vi "create channel offsets.vi"(7 "channelControl":T1(array[cluster]), 8 "offsets in":dbl[](array[numeric]), 9 "Offset to value:":dbl, 10 "Channel to match:":u16, 11 "Offset type:":T2(ring)) -> (0 "offsets out":dbl[](array[numeric]), 4 "updatedChannels":T1(array[cluster]))   [LabVIEW 2018]
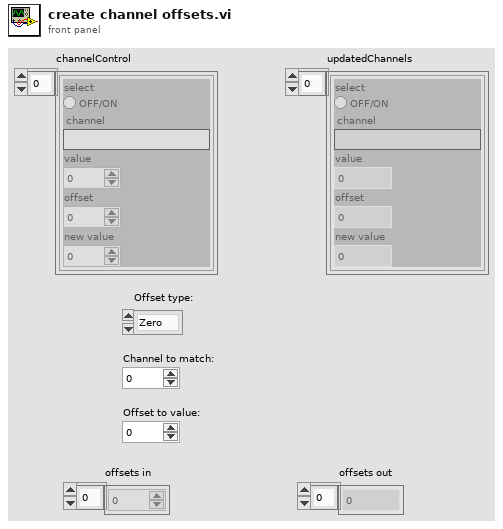
[diagram p1: front panel]
types:
  T1 = cluster{"select":bool, "channel":string, "value":dbl, "offset":dbl, "new value":dbl}[]
  T2 = enum16{"Zero", "Offset to value", "Offset to match channel", "Remove offset"}
  T3 = cluster{"select":bool, "channel":string, "value":dbl, "offset":dbl, "new value":dbl}
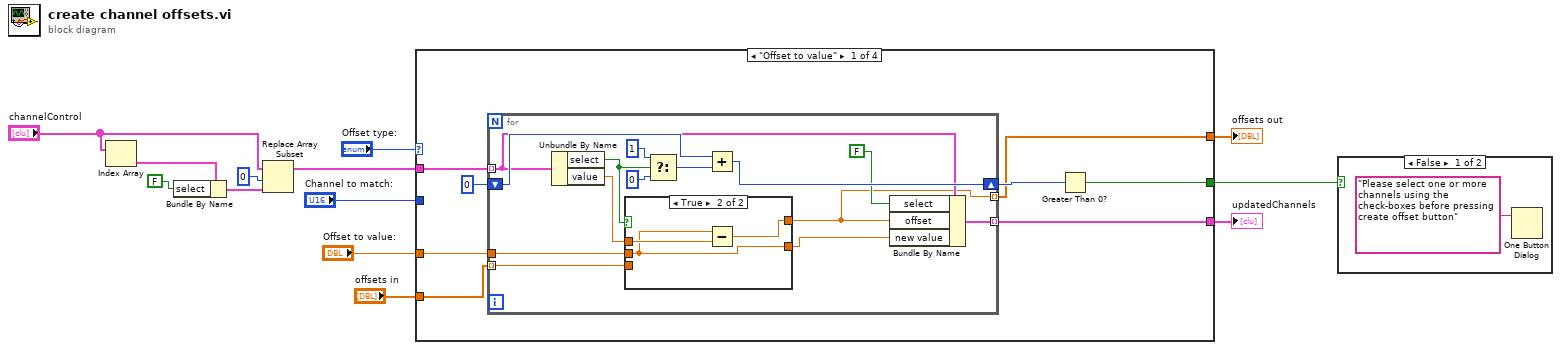
[diagram p0: block diagram]
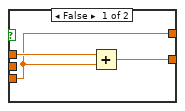
[diagram p3: hidden frame]
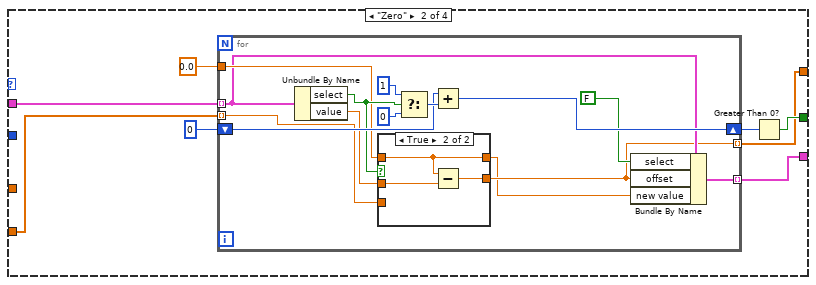
[diagram p4: hidden frame]
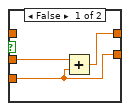
[diagram p5: hidden frame]
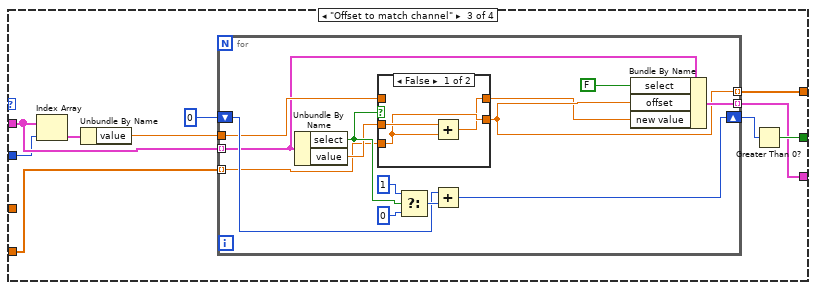
[diagram p6: hidden frame]
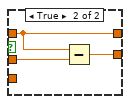
[diagram p7: hidden frame]
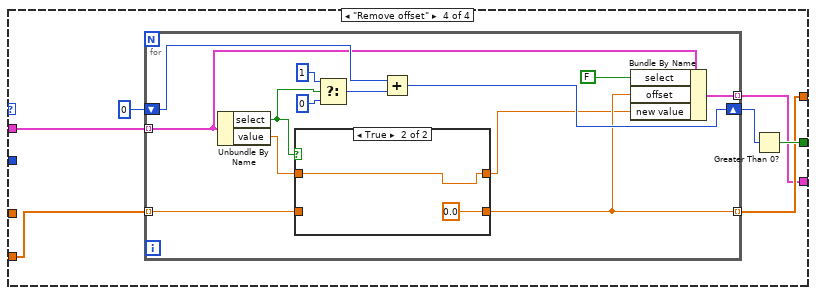
[diagram p8: hidden frame]
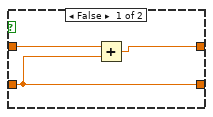
[diagram p9: hidden frame]
diagram:
  n1 = Index Array(array="channelControl") -> (element=w5:T3)  [unwired: 1 in]
  n2 = Bundle By Name(cluster=w5, "select"=FALSE) -> (w4:T3)
  n3 = Replace Array Subset(array="channelControl", new element=w4, index=0) -> (w7:T1)
  n4 = case shown="\"Offset to value\"" "Offset type:" {
    tunnel: "Offset to value:" -> [w16 _ _ _]
    tunnel: "Channel to match:" -> [_ _ w72 _]
    tunnel: [w15 w44 w75 w102] -> w9
    tunnel: "offsets in" -> [w19 w47 w78 w105]
    tunnel: w7 -> [w20 w48 w73 w100]
    tunnel: [w17 w45 w76 w103] -> w2
    tunnel: [w14 w43 w74 w101] -> w1
    frame "Offset to value" {
      n5 = for {
        shift-right: [w31] -> w18
        shift-left: 0 -> [w34]
        tunnel: w20 -> [w26] mode=indexing
        tunnel: w19 -> [w27] mode=indexing
        tunnel: w16 -> [w28]
        tunnel: [w23] -> w15 mode=indexing
        tunnel: [w25] -> w14 mode=indexing
        n6 = Unbundle By Name(w26) -> ("select"=w30:bool, "value"=w29:dbl)
        n7 = case shown="True" w30 {
          tunnel: w29 -> [w38 w41]
          tunnel: w28 -> [_ w39]
          tunnel: w27 -> [w37 _]
          tunnel: [w37 w40] -> w23
          tunnel: [w36 w39] -> w22
          frame False {
            n8 = Add(x=w38, y=w37) -> (x+y=w36:dbl)
          }
          frame True {
            n9 = Subtract(x=w39, y=w41) -> (x-y=w40:dbl)
          }
        }
        n10 = Select(t=1, s=w30, f=0) -> (s? t:f=w35:i32)
        n11 = Add(x=w34, y=w35) -> (x+y=w31:i32)
        n12 = Bundle By Name(cluster=w26, "select"=FALSE, "offset"=w23, "new value"=w22) -> (w25:T3)
      }
      n13 = Greater Than 0?(x=w18) -> (x > 0?=w17:bool)
    }
    frame "Zero" {
      n14 = for {
        shift-right: [w59] -> w46
        shift-left: 0 -> [w62]
        tunnel: w48 -> [w54] mode=indexing
        tunnel: w47 -> [w55] mode=indexing
        tunnel: 0.0 ("Offset to value:") -> [w56]
        tunnel: [w51] -> w44 mode=indexing
        tunnel: [w53] -> w43 mode=indexing
        n15 = Unbundle By Name(w54) -> ("select"=w58:bool, "value"=w57:dbl)
        n16 = case shown="True" w58 {
          tunnel: w57 -> [w66 w69]
          tunnel: w56 -> [_ w67]
          tunnel: w55 -> [w65 _]
          tunnel: [w65 w68] -> w51
          tunnel: [w64 w67] -> w50
          frame False {
            n17 = Add(x=w66, y=w65) -> (x+y=w64:dbl)
          }
          frame True {
            n18 = Subtract(x=w67, y=w69) -> (x-y=w68:dbl)
          }
        }
        n19 = Select(t=1, s=w58, f=0) -> (s? t:f=w63:i32)
        n20 = Add(x=w62, y=w63) -> (x+y=w59:i32)
        n21 = Bundle By Name(cluster=w54, "select"=FALSE, "offset"=w51, "new value"=w50) -> (w53:T3)
      }
      n22 = Greater Than 0?(x=w46) -> (x > 0?=w45:bool)
    }
    frame "Offset to match channel" {
      n23 = Index Array(array=w73, index=w72) -> (element=w71:T3)
      n24 = Unbundle By Name(w71) -> ("value"=w70:dbl)
      n25 = for {
        shift-right: [w89] -> w77
        shift-left: 0 -> [w92]
        tunnel: w73 -> [w84] mode=indexing
        tunnel: w78 -> [w85] mode=indexing
        tunnel: w70 -> [w86]
        tunnel: [w81] -> w75 mode=indexing
        tunnel: [w83] -> w74 mode=indexing
        n26 = Unbundle By Name(w84) -> ("select"=w88:bool, "value"=w87:dbl)
        n27 = case shown="False" w88 {
          tunnel: w87 -> [w96 w99]
          tunnel: w86 -> [_ w97]
          tunnel: w85 -> [w95 _]
          tunnel: [w95 w98] -> w81
          tunnel: [w94 w97] -> w80
          frame False {
            n28 = Add(x=w96, y=w95) -> (x+y=w94:dbl)
          }
          frame True {
            n29 = Subtract(x=w97, y=w99) -> (x-y=w98:dbl)
          }
        }
        n30 = Select(t=1, s=w88, f=0) -> (s? t:f=w93:i32)
        n31 = Add(x=w92, y=w93) -> (x+y=w89:i32)
        n32 = Bundle By Name(cluster=w84, "select"=FALSE, "offset"=w81, "new value"=w80) -> (w83:T3)
      }
      n33 = Greater Than 0?(x=w77) -> (x > 0?=w76:bool)
    }
    frame "Remove offset" {
      n34 = for {
        shift-right: [w115] -> w104
        shift-left: 0 -> [w118]
        tunnel: w100 -> [w111] mode=indexing
        tunnel: w105 -> [w112] mode=indexing
        tunnel: [w108] -> w102 mode=indexing
        tunnel: [w110] -> w101 mode=indexing
        n35 = Unbundle By Name(w111) -> ("select"=w114:bool, "value"=w113:dbl)
        n36 = case shown="True" w114 {
          tunnel: w113 -> [w122 w124]
          tunnel: w112 -> [w121 _]
          tunnel: [w121 0.0 ("value")] -> w108
          tunnel: [w120 w124] -> w107
          frame False {
            n37 = Add(x=w122, y=w121) -> (x+y=w120:dbl)
          }
          frame True {
          }
        }
        n38 = Select(t=1, s=w114, f=0) -> (s? t:f=w119:i32)
        n39 = Add(x=w118, y=w119) -> (x+y=w115:i32)
        n40 = Bundle By Name(cluster=w111, "select"=FALSE, "offset"=w108, "new value"=w107) -> (w110:T3)
      }
      n41 = Greater Than 0?(x=w104) -> (x > 0?=w103:bool)
    }
  }
  "offsets out" <- w9
  "updatedChannels" <- w1
  n42 = case shown="False" w2 {
    frame False {
      n43 = One Button Dialog(message="Please select one or more channels using the check-boxes before pressing create offset button") -> ()  [unwired: 1 in, 1 out]
    }
    frame True {
    }
  }
